vi "line to strings.vi"(11 "line":T1) -> (3 "strings":string[](array[string]))   [LabVIEW 2014, in "io editor node.lvclass"]
uses:
  io editor node.lvclass
  table line.ctl
  <vilib>/NI/Tag Bus Module Framework/channel/TBM channel.lvclass
  source/fifo channel/fifo channel.lvclass
  <vilib>/NI/Tag Bus/tag/tag descriptor.lvclass/tag descriptor.ctl
  <vilib>/NI/Tag Bus Module Framework/channel/TBM channel.lvclass/TBM channel.ctl
  source/fifo channel/fifo channel.lvclass/fifo channel.ctl
  source/fifo channel/Read fifo config.vi
  <vilib>/NI/Tag Bus/tag/read tag name.vi
  <vilib>/NI/Tag Bus Module Framework/channel/Read channel classification.vi
  <vilib>/NI/Tag Bus/tag/read data type.vi
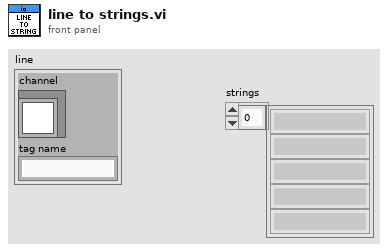
[diagram p1: front panel]
types:
  T1 = typedef "io editor node.lvclass/table line.ctl" = cluster{"channel":refnum<class "TBM channel.lvclass">, "tag name":string}
  T2 = typedef "TBM channel.lvclass/channel classification.ctl" = enum16{"input data", "output data", "processing parameter", "processing result"}
  T3 = typedef "tag bus.lvlib/tag descriptor.lvclass/Data Type.ctl" = enum16{"Double", "Single", "I64", "I32", "I16", "I8", "U64", "U32", "U16", "U8", "Boolean", "String", "Array of Double", "Array of Single", "Array of I64", "Array of I32", "Array of I16", "Array of I8", "Array of U64", "Array of U32", "Array of U16", "Array of U8", "Array of Boolean", "Array of String"}
  T4 = typedef "fifo channel.lvclass/fifo channel settings.ctl" = cluster{"Timeout":string, "Reset":string, "Averages":i32, "Samples":u32, "Channels":i32, "Fifo size":u32}
  T5 = typedef "io editor node.lvclass/permissions.ctl" = enum32{"Read from Indicator", "Write to Control"}
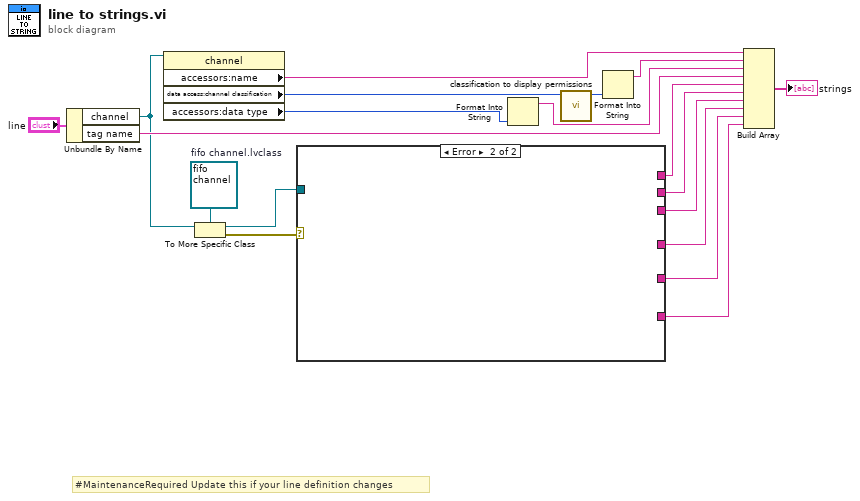
[diagram p0: block diagram]
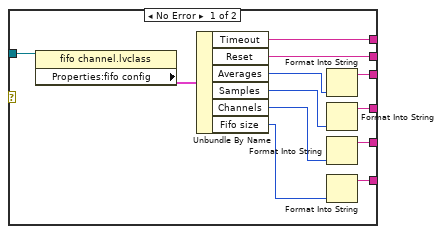
[diagram p2: hidden frame]
diagram:
  w10 = refnum<class "fifo channel.lvclass"> refnum  # fifo channel.lvclass
  # "#MaintenanceRequired Update this if your line definition changes"
  n1 = Unbundle By Name("line") -> ("channel"=w9:refnum<class "TBM channel.lvclass">, "tag name"=w13:string)
  n2 = property class="channel"(reference=w9) -> ("accessors:name"=w14:string, "data access:channel classification"=w15:T2, "accessors:data type"=w12:T3)  [unwired: 1 in, 2 out]
  n3 = To More Specific Class(target class=w10, reference=w9) -> (specific class reference=w7:refnum<class "fifo channel.lvclass">, error out=w8:errorcluster)  [unwired: 1 in]
  n4 = case shown="Error" w8 {
    tunnel: w7 -> [w31 _]
    tunnel: [w29 _] -> w6
    tunnel: [w28 _] -> w5
    tunnel: [w26 _] -> w4
    tunnel: [w24 _] -> w3
    tunnel: [w22 _] -> w2
    tunnel: [w20 _] -> w1
    frame No Error {
      n5 = property class="fifo channel.lvclass"(reference=w31) -> ("Properties:fifo config"=w30:T4)  [unwired: 1 in, 2 out]
      n6 = Unbundle By Name(w30) -> ("Timeout"=w29:string, "Reset"=w28:string, "Averages"=w27:i32, "Samples"=w25:u32, "Channels"=w23:i32, "Fifo size"=w21:u32)
      n7 = Format Into String(w27) -> (resulting string=w26:string)  [unwired: 3 in, 1 out]
      n8 = Format Into String(w25) -> (resulting string=w24:string)  [unwired: 3 in, 1 out]
      n9 = Format Into String(w23) -> (resulting string=w22:string)  [unwired: 3 in, 1 out]
      n10 = Format Into String(w21) -> (resulting string=w20:string)  [unwired: 3 in, 1 out]
    }
    frame Error {
    }
  }
  n11 = Format Into String(w12) -> (resulting string=w11:string)  [unwired: 3 in, 1 out]
  n12 = call "classification to display permissions.vi"("channel classification"=w15) -> ("permissions"=w17:T5)  [unwired: 10 in]
  n13 = Format Into String(w17) -> (resulting string=w16:string)  [unwired: 3 in, 1 out]
  n14 = Build Array(w14, w16, w11, w13, w6, w5, w4, w3, w2, w1) -> (→"strings":string[])
